vi "PLC.Debug.Simulator.vi"() -> ()   [LabVIEW 2016]
uses:
  Database/Database.Global.vi
  LowLevel/PLC.DataBlock.PLCchangeover.ctl
  LowLevel/PLC.DataBlock.PCchangeover.ctl
  LowLevel/PLC.DataBlock.PLCcheckstatus.ctl
  <vilib>/Utility/miscctls.llb/LVPointTypeDef.ctl
  LowLevel/PLC.DataBlock.PCcheckstatus.ctl
panel:
  in  "NewDataContinuous":bool caption="Status"
  out "_loop":i32(ring)=4
  in  "NewDataSingle":bool caption="Status"
  in  "NewDataComponentBAM":string="3000000" caption="Component BAM"
  in  "NewDataComponentHousing":string="2000000" caption="Component Housing"
  in  "NewDataProductSerial":string="1000000" caption="Product Serial"
  out "PLCcheckstatus":T1
  in  "CheckComponentSerial":string caption="Component Serial"
  out "PCcheckstatus":T2
  in  "CheckProductSerial":string caption="Product Serial"
  in  "CheckStatus":bool caption="Status"
  in  "CheckStation":i32(ring) caption="Station" items=["AS_010.01.A_cTCV", "AS_010.01.B_cTCV", "AS_010.01.C_cTCV", "AS_020.01.A_cTCV", "AS_030.01.A_cTCV", "AS_030.01.B_cTCV", "AS_040.01.A_cTCV", "AS_050.01.A_cTCV", "AS_060.01.A_cTCV", "AS_060.01.B_cTCV", "AS_060.01.C_cTCV", "AS_070.01.A_cTCV", "AS_070.02.A_cTCV", "AS_070.01.B_cTCV", "TB_071.01.A_cTCV", "AS_080.01.A_cTCV"]
  out "PCchangeover":T3 caption="AS_030.01.A_cTCV" {"TVH" format="%.3f"; "TVL" format="%.3f"; "TP" format="%.3f"}
  out "Variant.Refs":refnum<vi>[](array[refnum])
  in  "Variant BAM":u16(ring) caption="BAM" items=["", "9998887773"]
  in  "Variant Housing":u16(ring) caption="Housing" items=["", "9998887772"]
  in  "Variant ProdLine":u16(ring) caption="Main" items=["", "9998887770", "9998887771"]
  in  "Variant 15":u16(ring) caption="AS_080.01.A_cTCV" items=["", "9998887770", "9998887771"]
  in  "Variant 03":u16(ring) caption="AS_020.01.A_cTCV" items=["", "9998887770", "9998887771"]
  in  "Variant 14":u16(ring) caption="TB_071.01.A_cTCV" items=["", "9998887770", "9998887771"]
  in  "Variant 13":u16(ring) caption="AS_070.01.B_cTCV" items=["", "9998887770"]
  in  "Variant 12":u16(ring) caption="AS_070.02.A_cTCV" items=["", "9998887771"]
  in  "Variant 11":u16(ring) caption="AS_070.01.A_cTCV" items=["", "9998887770"]
  in  "Variant 10":u16(ring) caption="AS_060.01.C_cTCV" items=["", "9998887773"]
  in  "Variant 09":u16(ring) caption="AS_060.01.B_cTCV" items=["", "9998887773"]
  in  "Variant 08":u16(ring) caption="AS_060.01.A_cTCV" items=["", "9998887773"]
  in  "Variant 07":u16(ring) caption="AS_050.01.A_cTCV" items=["", "9998887770"]
  in  "Variant 06":u16(ring) caption="AS_040.01.A_cTCV" items=["", "9998887770", "9998887771"]
  in  "Variant 05":u16(ring) caption="AS_030.01.B_cTCV" items=["", "9998887772"]
  in  "Variant 04":u16(ring) caption="AS_030.01.A_cTCV" items=["", "9998887772"]
  in  "Variant 02":u16(ring) caption="AS_010.01.C_cTCV" items=["", "9998887770"]
  in  "Variant 01":u16(ring) caption="AS_010.01.B_cTCV" items=["", "9998887770", "9998887771"]
  in  "Variant 00":u16(ring) caption="AS_010.01.A_cTCV" items=["", "9998887770", "9998887771"]
  out "ChangeoverData":T3[](array[typedef]) {"TVH" format="%.3f"; "TVL" format="%.3f"; "TP" format="%.3f"}
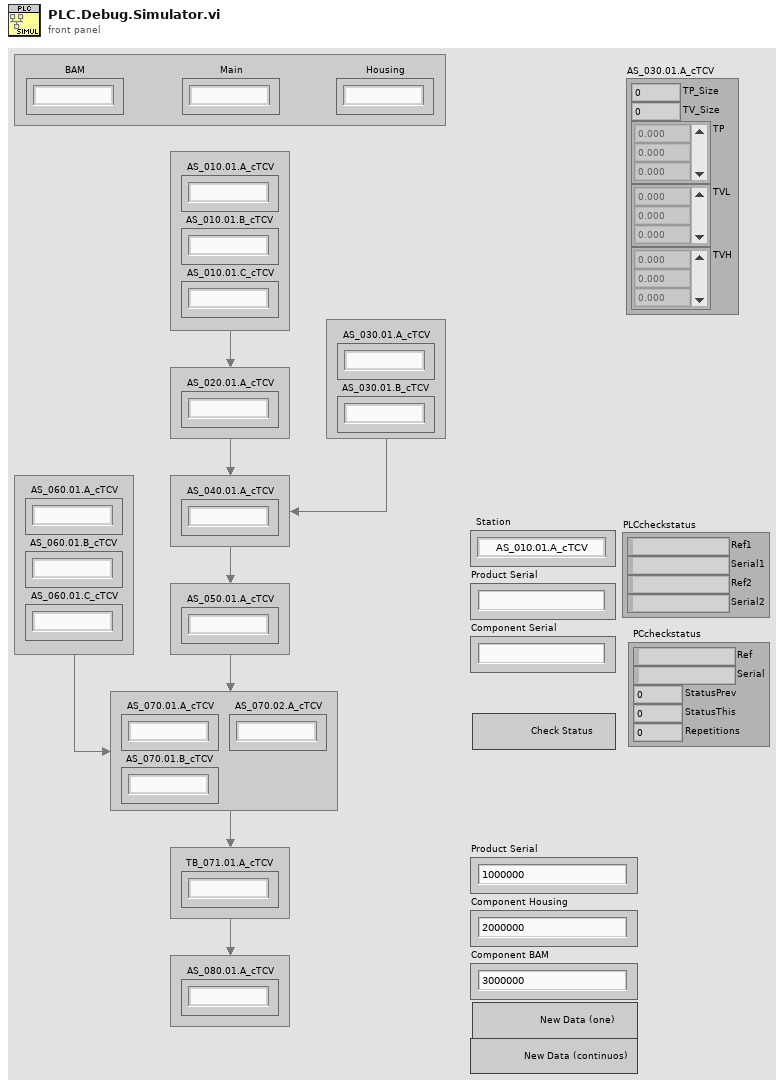
[diagram p1: front panel]
types:
  T1 = typedef "PLC.DataBlock.PLCcheckstatus.ctl" = cluster{"Ref1":string, "Serial1":string, "Ref2":string, "Serial2":string}
  T2 = typedef "PLC.DataBlock.PCcheckstatus.ctl" = cluster{"Ref":string, "Serial":string, "StatusPrev":i8, "StatusThis":i8, "Repetitions":u8}
  T3 = typedef "PLC.DataBlock.PCchangeover.ctl" = cluster{"TP_Size":u8, "TV_Size":u8, "TP":sgl[], "TVL":sgl[], "TVH":sgl[]}
  T4 = typedef "LVPointTypeDef.ctl" = cluster{"Horizontal":i16, "Vertical":i16}
  T5 = enum8{"Enabled", "Disabled", "Disabled and Grayed Out"}
  T6 = typedef "PLC.DataBlock.PLCchangeover.ctl" = cluster{"Ref":string}
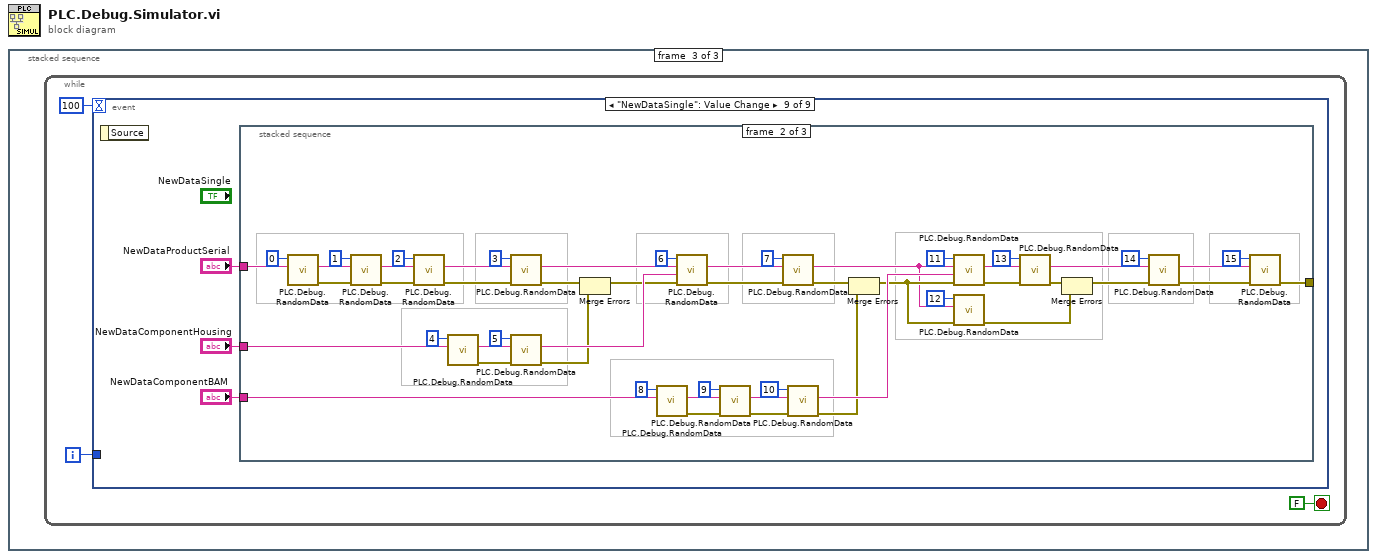
[diagram p0: block diagram]
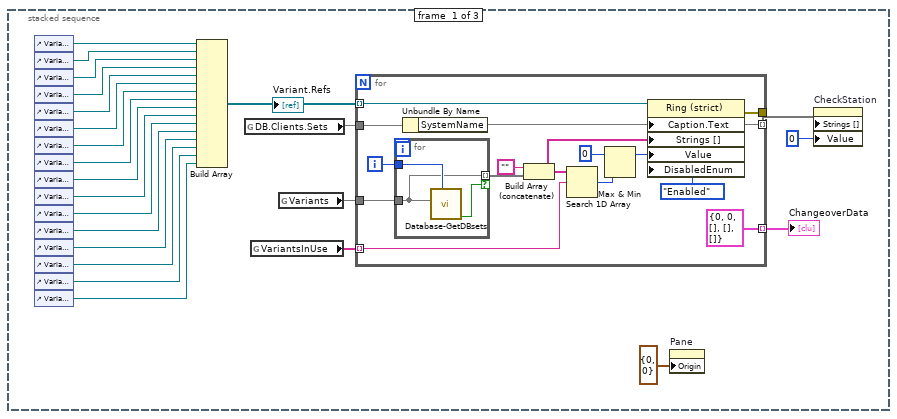
[diagram p2: hidden frame]
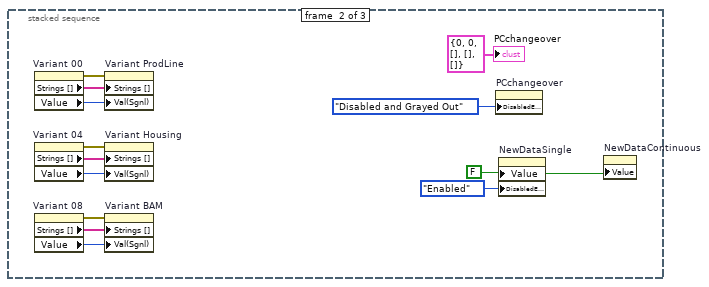
[diagram p3: hidden frame]
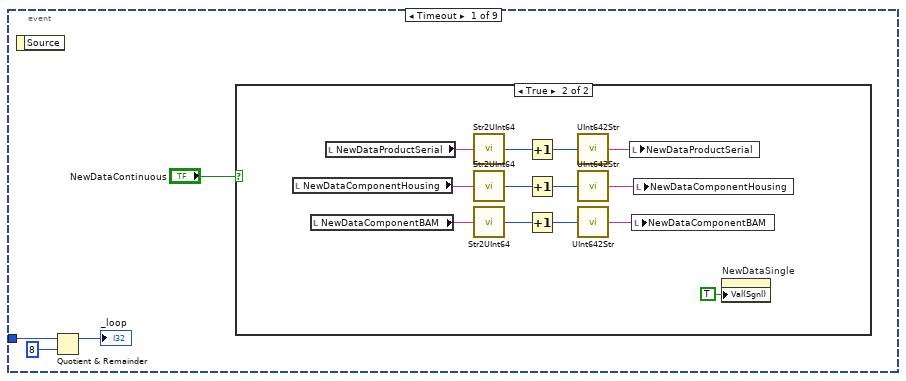
[diagram p4: hidden frame]
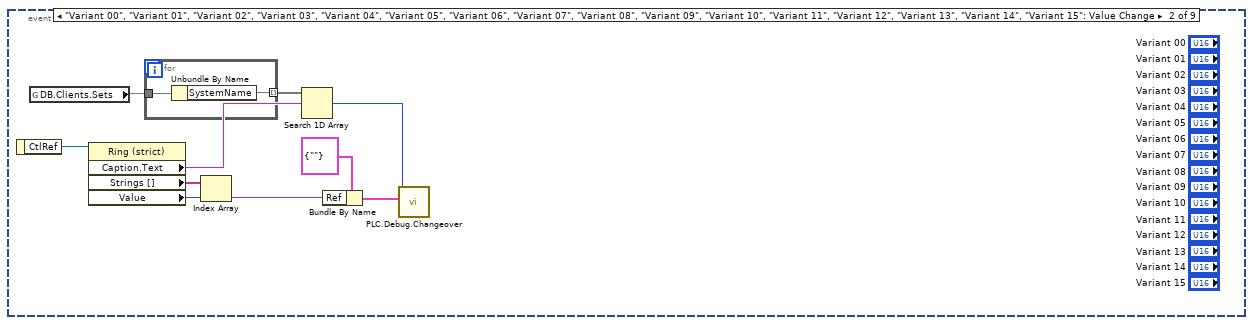
[diagram p6: hidden frame]
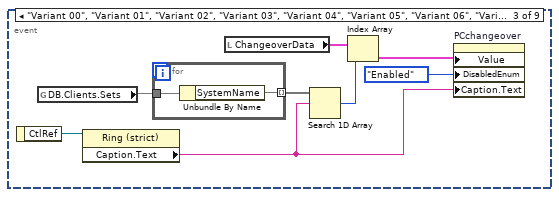
[diagram p7: hidden frame]
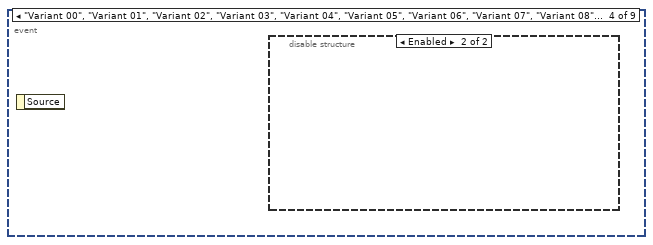
[diagram p8: hidden frame]
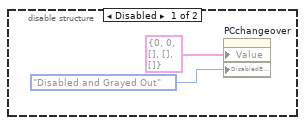
[diagram p9: hidden frame]
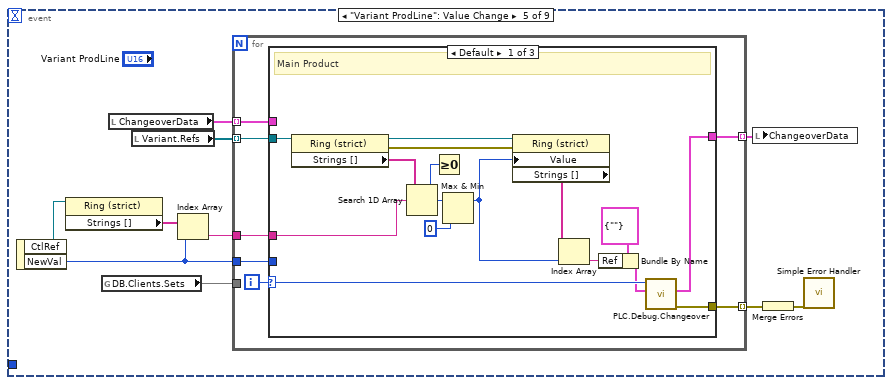
[diagram p10: hidden frame]
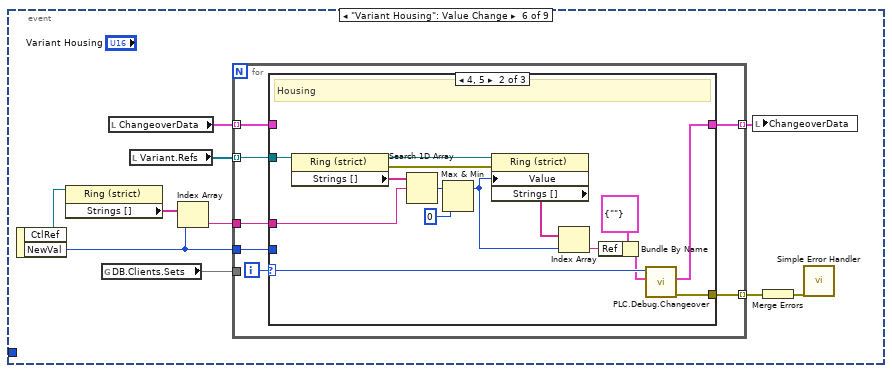
[diagram p13: hidden frame]
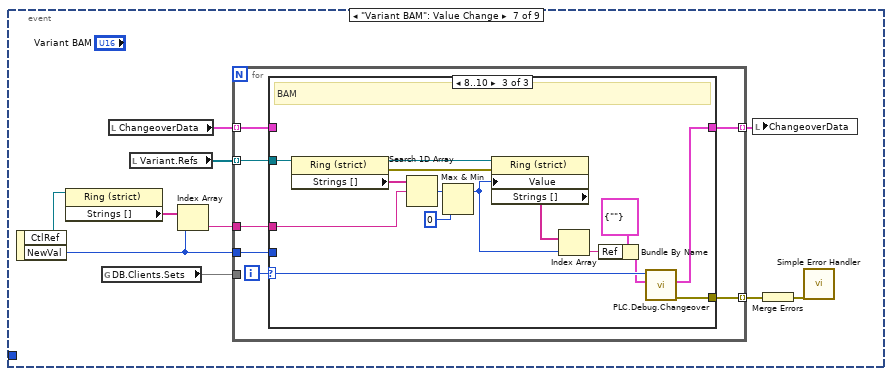
[diagram p16: hidden frame]
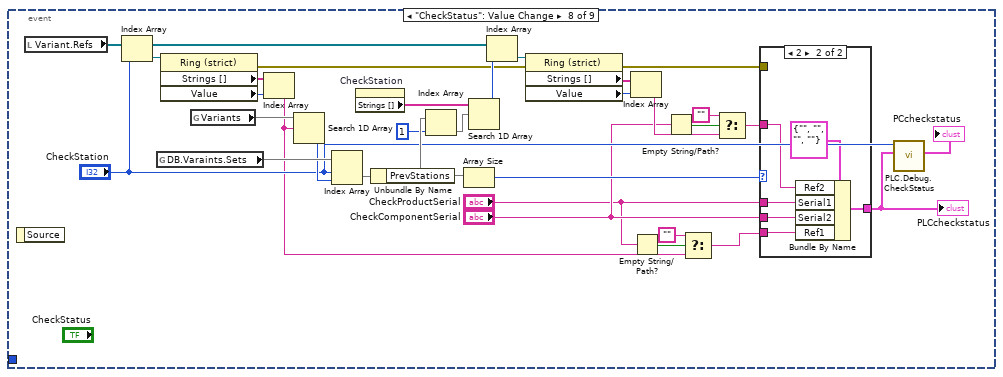
[diagram p19: hidden frame]
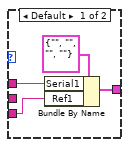
[diagram p20: hidden frame]
diagram:
  n1 = stacked-sequence {
    frame #0 {
      n2 = control-ref of="Variant 00"() -> (w7:refnum<vi>)
      n3 = control-ref of="Variant 01"() -> (w8:refnum<vi>)
      n4 = control-ref of="Variant 02"() -> (w9:refnum<vi>)
      n5 = control-ref of="Variant 03"() -> (w10:refnum<vi>)
      n6 = control-ref of="Variant 04"() -> (w11:refnum<vi>)
      n7 = control-ref of="Variant 05"() -> (w12:refnum<vi>)
      n8 = control-ref of="Variant 06"() -> (w13:refnum<vi>)
      n9 = control-ref of="Variant 07"() -> (w14:refnum<vi>)
      n10 = control-ref of="Variant 08"() -> (w15:refnum<vi>)
      n11 = control-ref of="Variant 09"() -> (w16:refnum<vi>)
      n12 = control-ref of="Variant 10"() -> (w17:refnum<vi>)
      n13 = control-ref of="Variant 11"() -> (w18:refnum<vi>)
      n14 = control-ref of="Variant 12"() -> (w19:refnum<vi>)
      n15 = control-ref of="Variant 13"() -> (w20:refnum<vi>)
      n16 = control-ref of="Variant 14"() -> (w21:refnum<vi>)
      n17 = control-ref of="Variant 15"() -> (w22:refnum<vi>)
      n18 = Build Array(w7, w8, w9, w10, w11, w12, w13, w14, w15, w16, w17, w18, w19, w20, w21, w22) -> (w6:refnum<vi>[])
      "Variant.Refs" <- w6
      n19 = global read "Database.Global.vi" "DB.Clients.Sets"() -> (w24)
      n20 = global read "Database.Global.vi" "VariantsInUse"() -> (w4:string[])
      n21 = global read "Database.Global.vi" "Variants"() -> (w23)
      n22 = for {
        tunnel: w24 -> [w37]
        tunnel: w23 -> [w39]
        tunnel: w6 -> [w33] mode=indexing
        tunnel: [w36] -> _
        tunnel: [T3 {"TP_Size"=0, "TV_Size"=0, "TP"=[], "TVL"=[], "TVH"=[]} ("PCchangeover")] -> w5 mode=indexing
        tunnel: w4 -> [w25] mode=indexing
        tunnel: [w26] -> w3 mode=indexing
        i -> [w38]
        n23 = for {
          tunnel: w39 -> [w41]
          tunnel: w38 -> [w42]
          tunnel: [w41] -> w35 mode=indexing if=w40
          n24 = call "Database-GetDBsets.vi"("Idx"=w42, "Variant"=w41) -> ("Found"=w40:bool)  [unwired: 5 in, 4 out]
        }
        n25 = Unbundle By Name(w37) -> ("SystemName"=w26)
        n26 = Build Array (concatenate)("", w35) -> (w28:string[])
        n27 = Search 1D Array(1D array=w28, element=w25) -> (index of element=w31:i32)  [unwired: 1 in]
        n28 = Max & Min(x=0 ("Value"), y=w31) -> (max(x,y)=w29:i32)  [unwired: 1 out]
        n29 = property class="Ring (strict)"(reference=w33, "Caption.Text"=w26, "Strings []"=w28, "Value"=w29, "DisabledEnum"=T5."Enabled" ("Disabled")) -> (error out=w36:errorcluster)  [unwired: 1 in, 1 out]
      }
      "ChangeoverData" <- w5
      n30 = property on="Pane" class="Pane"("Origin"=T4 {"Horizontal"=0, "Vertical"=0}) -> ()  [unwired: 2 in, 2 out]
      n31 = property on="CheckStation" class="Ring (strict)"("Strings []"=w3, "Value"=0) -> ()  [unwired: 2 in, 2 out]
    }
    frame #1 {
      w43 = FALSE ("NewDataSingle")
      n32 = property on="Variant 00" class="Ring (strict)"() -> (error out=w52:errorcluster, "Strings []"=w55:string[], "Value"=w47:u16)  [unwired: 2 in, 1 out]
      n33 = property on="Variant 04" class="Ring (strict)"() -> (error out=w51:errorcluster, "Strings []"=w54:string[], "Value"=w48:u16)  [unwired: 2 in, 1 out]
      n34 = property on="Variant 08" class="Ring (strict)"() -> (error out=w50:errorcluster, "Strings []"=w53:string[], "Value"=w49:u16)  [unwired: 2 in, 1 out]
      n35 = property on="Variant ProdLine" class="Ring (strict)"(error in=w52, "Strings []"=w55, "Val(Sgnl)"=w47) -> ()  [unwired: 1 in, 2 out]
      n36 = property on="Variant Housing" class="Ring (strict)"(error in=w51, "Strings []"=w54, "Val(Sgnl)"=w48) -> ()  [unwired: 1 in, 2 out]
      n37 = property on="Variant BAM" class="Ring (strict)"(error in=w50, "Strings []"=w53, "Val(Sgnl)"=w49) -> ()  [unwired: 1 in, 2 out]
      n38 = property on="PCchangeover" class="Clust (strict)"("DisabledEnum"=T5."Disabled and Grayed Out" ("Disabled")) -> ()  [unwired: 2 in, 2 out]
      n39 = property on="NewDataSingle" class="Bool (strict)"("Value"=w43, "DisabledEnum"=T5."Enabled" ("Disabled")) -> ()  [unwired: 2 in, 2 out]
      n40 = property on="NewDataContinuous" class="Bool (strict)"("Value"=w43) -> ()  [unwired: 2 in, 2 out]
      "PCchangeover" <- T3 {"TP_Size"=0, "TV_Size"=0, "TP"=[], "TVL"=[], "TVH"=[]} ("PCchangeover")
    }
    frame #2 {
      n41 = while {
        i -> [w56]
        stop <- FALSE stop-if-true
        n42 = event shown="[8] \"NewDataSingle\": Value Change" {
          selector: _ -> [_ _ _ _ _ _ _ _ _]
          dyn-events: _ -> [_ _ _ _ _ _ _ _ _]
          timeout: 100 -> [_ _ _ _ _ _ _ _ _]
          tunnel: w56 -> [w60 _ _ _ _ _ _ _ _]
          event Timeout {
            n43 = event-data() -> ()  [unwired: 1 in, 1 out]
            n44 = Quotient & Remainder(x=w60, y=8) -> (x-y*floor(x/y)=→"_loop":i32)  [unwired: 1 out]
            n45 = case shown="True" "NewDataContinuous" {
              frame False {
              }
              frame True {
                n46 = local read "NewDataComponentHousing"() -> (w70:string)
                n47 = local read "NewDataComponentBAM"() -> (w65:string)
                n48 = local read "NewDataProductSerial"() -> (w73:string)
                n49 = call "Str2UInt64.vi"("string"=w73) -> ("Numeric"=w74:u64)
                n50 = call "Str2UInt64.vi"("string"=w70) -> ("Numeric"=w69:u64)
                n51 = call "Str2UInt64.vi"("string"=w65) -> ("Numeric"=w66:u64)
                n52 = Increment(x=w74) -> (x+1=w72:u64)
                n53 = Increment(x=w69) -> (x+1=w71:u64)
                n54 = Increment(x=w66) -> (x+1=w64:u64)
                n55 = call "UInt642Str.vi"("Numeric"=w72) -> ("string"=w75:string)
                n56 = call "UInt642Str.vi"("Numeric"=w71) -> ("string"=w68:string)
                n57 = call "UInt642Str.vi"("Numeric"=w64) -> ("string"=w67:string)
                n58 = local write "NewDataProductSerial"(w75) -> ()
                n59 = local write "NewDataComponentBAM"(w67) -> ()
                n60 = local write "NewDataComponentHousing"(w68) -> ()
                n61 = property on="NewDataSingle" class="Bool (strict)"("Val(Sgnl)"=TRUE ("Value (Signaling)")) -> ()  [unwired: 2 in, 2 out]
              }
            }
          }
          event "Variant 00", "Variant 01", "Variant 02", "Variant 03", "Variant 04", "Variant 05", "Variant 06", "Variant 07", "Variant 08", "Variant 09", "Variant 10", "Variant 11", "Variant 12", "Variant 13", "Variant 14", "Variant 15": Value Change {
            n62 = event-data() -> ("CtlRef"=w85:refnum<vi>)  [unwired: 1 in]
            n63 = global read "Database.Global.vi" "DB.Clients.Sets"() -> (w79)
            n64 = property class="Ring (strict)"(reference=w85) -> ("Caption.Text"=w77:string, "Strings []"=w82:string[], "Value"=w83:u16)  [unwired: 1 in, 2 out]
            n65 = for {
              tunnel: w79 -> [w87]
              tunnel: [w86] -> w78 mode=indexing
              n66 = Unbundle By Name(w87) -> ("SystemName"=w86)
            }
            n67 = Index Array(array=w82, index=w83) -> (element=w81:string)
            n68 = Search 1D Array(1D array=w78, element=w77) -> (index of element=w76:i32)  [unwired: 1 in]
            n69 = Bundle By Name(cluster=T6 {"Ref"=""} ("PLCchangeover"), "Ref"=w81) -> (w80:T6)
            n70 = call "PLC.Debug.Changeover.vi"("PLCchangeover"=w80, "Idx"=w76) -> ()  [unwired: 8 in, 2 out]
          }
          event "Variant 00", "Variant 01", "Variant 02", "Variant 03", "Variant 04", "Variant 05", "Variant 06", "Variant 07", "Variant 08", "Variant 09", "Variant 10", "Variant 12", "Variant 13", "Variant 14", "Variant 15": Mouse Enter {
            n71 = event-data() -> ("CtlRef"=w95:refnum<vi>)  [unwired: 1 in]
            n72 = global read "Database.Global.vi" "DB.Clients.Sets"() -> (w92)
            n73 = property class="Ring (strict)"(reference=w95) -> ("Caption.Text"=w88:string)  [unwired: 1 in, 2 out]
            n74 = for {
              tunnel: w92 -> [w97]
              tunnel: [w96] -> w91 mode=indexing
              n75 = Unbundle By Name(w97) -> ("SystemName"=w96)
            }
            n76 = local read "ChangeoverData"() -> (w94:T3[])
            n77 = Search 1D Array(1D array=w91, element=w88) -> (index of element=w90:i32)  [unwired: 1 in]
            n78 = Index Array(array=w94, index=w90) -> (element=w93:T3)
            n79 = property on="PCchangeover" class="Clust (strict)"("Value"=w93, "DisabledEnum"=T5."Enabled" ("Disabled"), "Caption.Text"=w88) -> ()  [unwired: 2 in, 2 out]
          }
          event "Variant 00", "Variant 01", "Variant 02", "Variant 03", "Variant 04", "Variant 05", "Variant 06", "Variant 07", "Variant 08", "Variant 09", "Variant 10", "Variant 11", "Variant 12", "Variant 13", "Variant 14", "Variant 15": Mouse Leave {
            n80 = event-data() -> ()  [unwired: 1 in, 1 out]
            n81 = disable-structure shown="Enabled" {
              frame Disabled {
                n82 = property on="PCchangeover" class="Clust (strict)"("Value"=T3 {"TP_Size"=0, "TV_Size"=0, "TP"=[], "TVL"=[], "TVH"=[]} ("PCchangeover"), "DisabledEnum"=T5."Disabled and Grayed Out" ("Disabled")) -> ()  [unwired: 2 in, 2 out]
              }
              frame Enabled {
              }
            }
          }
          event "Variant ProdLine": Value Change {
            n83 = event-data() -> ("CtlRef"=w101:refnum<vi>, "NewVal"=w102:u16)  [unwired: 1 in]
            n84 = property class="Ring (strict)"(reference=w101) -> ("Strings []"=w103:string[])  [unwired: 1 in, 2 out]
            n85 = global read "Database.Global.vi" "DB.Clients.Sets"() -> (w109)
            n86 = local read "ChangeoverData"() -> (w105:T3[])
            n87 = local read "Variant.Refs"() -> (w106:refnum<vi>[])
            n88 = Index Array(array=w103, index=w102) -> (element=w100:string)
            n89 = for {
              tunnel: w109 -> [_]
              tunnel: w106 -> [w111] mode=indexing
              tunnel: w102 -> [w115]
              tunnel: [w114] -> w108 mode=indexing
              tunnel: w105 -> [w113] mode=indexing
              tunnel: [w112] -> w104 mode=indexing
              tunnel: w100 -> [w110]
              i -> [w116]
              n90 = case shown="Default" w116 {
                selector: w116 -> [w129 _ _]
                tunnel: w111 -> [w125 _ _]
                tunnel: w115 -> [_ _ _]
                tunnel: [w127 _ _] -> w114
                tunnel: w113 -> [_ w132 w133]
                tunnel: [w126 w132 w133] -> w112
                tunnel: w110 -> [w122 _ _]
                frame Default {
                  # "Main Product"
                  n91 = property class="Ring (strict)"(reference=w125) -> (reference out=w124:refnum<vi>, error out=w120:errorcluster, "Strings []"=w123:string[])  [unwired: 1 in]
                  n92 = Search 1D Array(1D array=w123, element=w122) -> (index of element=w117:i32)  [unwired: 1 in]
                  n93 = Greater Or Equal To 0?(x=w117) -> ()  [unwired: 1 out]
                  n94 = Max & Min(x=w117, y=0) -> (max(x,y)=w118:i32)  [unwired: 1 out]
                  n95 = property class="Ring (strict)"(reference=w124, error in=w120, "Value"=w118) -> ("Strings []"=w119:string[])  [unwired: 2 out]
                  n96 = Index Array(array=w119, index=w118) -> (element=w130:string)
                  n97 = Bundle By Name(cluster=T6 {"Ref"=""} ("PLCchangeover"), "Ref"=w130) -> (w128:T6)
                  n98 = call "PLC.Debug.Changeover.vi"("PLCchangeover"=w128, "Idx"=w129) -> ("error out"=w127:errorcluster, "PCchangeover"=w126:T3)  [unwired: 8 in]
                }
                frame 4, 5 {
                  # "Housing"
                }
                frame 8..10 {
                  # "BAM"
                }
              }
            }
            n99 = local write "ChangeoverData"(w104) -> ()
            n100 = Merge Errors(w108) -> (w107:errorcluster)
            n101 = call <vilib>:"Simple Error Handler.vi"("error in (no error)"=w107) -> ()  [unwired: 4 in, 5 out]
          }
          event "Variant Housing": Value Change {
            n102 = event-data() -> ("CtlRef"=w135:refnum<vi>, "NewVal"=w136:u16)  [unwired: 1 in]
            n103 = property class="Ring (strict)"(reference=w135) -> ("Strings []"=w137:string[])  [unwired: 1 in, 2 out]
            n104 = global read "Database.Global.vi" "DB.Clients.Sets"() -> (w143)
            n105 = local read "ChangeoverData"() -> (w139:T3[])
            n106 = local read "Variant.Refs"() -> (w140:refnum<vi>[])
            n107 = Index Array(array=w137, index=w136) -> (element=w134:string)
            n108 = for {
              tunnel: w143 -> [_]
              tunnel: w140 -> [w145] mode=indexing
              tunnel: w136 -> [w149]
              tunnel: [w148] -> w142 mode=indexing
              tunnel: w139 -> [w147] mode=indexing
              tunnel: [w146] -> w138 mode=indexing
              tunnel: w134 -> [w144]
              i -> [w150]
              n109 = case shown="4, 5" w150 {
                selector: w150 -> [_ w164 _]
                tunnel: w145 -> [_ w160 _]
                tunnel: w149 -> [_ _ _]
                tunnel: [_ w162 _] -> w148
                tunnel: w147 -> [w151 _ w167]
                tunnel: [w151 w161 w167] -> w146
                tunnel: w144 -> [_ w157 _]
                frame Default {
                  # "Main Product"
                }
                frame 4, 5 {
                  # "Housing"
                  n110 = property class="Ring (strict)"(reference=w160) -> (reference out=w159:refnum<vi>, error out=w154:errorcluster, "Strings []"=w158:string[])  [unwired: 1 in]
                  n111 = Search 1D Array(1D array=w158, element=w157) -> (index of element=w156:i32)  [unwired: 1 in]
                  n112 = Max & Min(x=w156, y=0) -> (max(x,y)=w152:i32)  [unwired: 1 out]
                  n113 = property class="Ring (strict)"(reference=w159, error in=w154, "Value"=w152) -> ("Strings []"=w153:string[])  [unwired: 2 out]
                  n114 = Index Array(array=w153, index=w152) -> (element=w165:string)
                  n115 = Bundle By Name(cluster=T6 {"Ref"=""} ("PLCchangeover"), "Ref"=w165) -> (w163:T6)
                  n116 = call "PLC.Debug.Changeover.vi"("PLCchangeover"=w163, "Idx"=w164) -> ("error out"=w162:errorcluster, "PCchangeover"=w161:T3)  [unwired: 8 in]
                }
                frame 8..10 {
                  # "BAM"
                }
              }
            }
            n117 = local write "ChangeoverData"(w138) -> ()
            n118 = Merge Errors(w142) -> (w141:errorcluster)
            n119 = call <vilib>:"Simple Error Handler.vi"("error in (no error)"=w141) -> ()  [unwired: 4 in, 5 out]
          }
          event "Variant BAM": Value Change {
            n120 = event-data() -> ("CtlRef"=w169:refnum<vi>, "NewVal"=w170:u16)  [unwired: 1 in]
            n121 = property class="Ring (strict)"(reference=w169) -> ("Strings []"=w171:string[])  [unwired: 1 in, 2 out]
            n122 = global read "Database.Global.vi" "DB.Clients.Sets"() -> (w177)
            n123 = local read "ChangeoverData"() -> (w173:T3[])
            n124 = local read "Variant.Refs"() -> (w174:refnum<vi>[])
            n125 = Index Array(array=w171, index=w170) -> (element=w168:string)
            n126 = for {
              tunnel: w177 -> [_]
              tunnel: w174 -> [w179] mode=indexing
              tunnel: w170 -> [w183]
              tunnel: [w182] -> w176 mode=indexing
              tunnel: w173 -> [w181] mode=indexing
              tunnel: [w180] -> w172 mode=indexing
              tunnel: w168 -> [w178]
              i -> [w184]
              n127 = case shown="8..10" w184 {
                selector: w184 -> [_ _ w199]
                tunnel: w179 -> [_ _ w195]
                tunnel: w183 -> [_ _ _]
                tunnel: [_ _ w197] -> w182
                tunnel: w181 -> [w185 w186 _]
                tunnel: [w185 w186 w196] -> w180
                tunnel: w178 -> [_ _ w192]
                frame Default {
                  # "Main Product"
                }
                frame 4, 5 {
                  # "Housing"
                }
                frame 8..10 {
                  # "BAM"
                  n128 = property class="Ring (strict)"(reference=w195) -> (reference out=w194:refnum<vi>, error out=w189:errorcluster, "Strings []"=w193:string[])  [unwired: 1 in]
                  n129 = Search 1D Array(1D array=w193, element=w192) -> (index of element=w191:i32)  [unwired: 1 in]
                  n130 = Max & Min(x=w191, y=0) -> (max(x,y)=w187:i32)  [unwired: 1 out]
                  n131 = property class="Ring (strict)"(reference=w194, error in=w189, "Value"=w187) -> ("Strings []"=w188:string[])  [unwired: 2 out]
                  n132 = Index Array(array=w188, index=w187) -> (element=w200:string)
                  n133 = Bundle By Name(cluster=T6 {"Ref"=""} ("PLCchangeover"), "Ref"=w200) -> (w198:T6)
                  n134 = call "PLC.Debug.Changeover.vi"("PLCchangeover"=w198, "Idx"=w199) -> ("error out"=w197:errorcluster, "PCchangeover"=w196:T3)  [unwired: 8 in]
                }
              }
            }
            n135 = local write "ChangeoverData"(w172) -> ()
            n136 = Merge Errors(w176) -> (w175:errorcluster)
            n137 = call <vilib>:"Simple Error Handler.vi"("error in (no error)"=w175) -> ()  [unwired: 4 in, 5 out]
          }
          event "CheckStatus": Value Change {
            n138 = event-data() -> ()  [unwired: 1 in, 1 out]
            n139 = local read "Variant.Refs"() -> (w214:refnum<vi>[])
            n140 = Index Array(array=w214, index="CheckStation") -> (element=w233:refnum<vi>)
            n141 = global read "Database.Global.vi" "DB.Varaints.Sets"() -> (w230)
            n142 = property class="Ring (strict)"(reference=w233) -> (error out=w213:errorcluster, "Strings []"=w231:string[], "Value"=w232:u16)  [unwired: 1 in, 1 out]
            n143 = global read "Database.Global.vi" "Variants"() -> (w222)
            n144 = Index Array(array=w231, index=w232) -> (element=w210:string)
            n145 = Search 1D Array(1D array=w222, element=w210) -> (index of element=w229:i32)  [unwired: 1 in]
            n146 = Index Array(array=w230, index (row)="CheckStation", index (col)=w229) -> (element=w228)
            n147 = property on="CheckStation" class="Ring (strict)"() -> ("Strings []"=w226:string[])  [unwired: 2 in, 2 out]
            n148 = Unbundle By Name(w228) -> ("PrevStations"=w225)
            n149 = Index Array(array=w225, index=1) -> (element=w220)
            n150 = Array Size(array=w225) -> (size(s)=w227:i32)
            n151 = Search 1D Array(1D array=w226, element=w220) -> (index of element=w223:i32)  [unwired: 1 in]
            n152 = Index Array(array=w214, index=w223) -> (element=w216:refnum<vi>)
            n153 = property class="Ring (strict)"(reference=w216, error in=w213) -> (error out=w215:errorcluster, "Strings []"=w219:string[], "Value"=w218:u16)  [unwired: 1 out]
            n154 = Index Array(array=w219, index=w218) -> (element=w205:string)
            n155 = Empty String/Path?(string/path="CheckProductSerial") -> (empty?=w211:bool)
            n156 = Empty String/Path?(string/path="CheckComponentSerial") -> (empty?=w207:bool)
            n157 = Select(t="", s=w211, f=w210) -> (s? t:f=w208:string)
            n158 = Select(t="", s=w207, f=w205) -> (s? t:f=w204:string)
            n159 = case shown="2" w227 {
              tunnel: [w237 w243] -> w221
              tunnel: w208 -> [w236 w242]
              tunnel: "CheckProductSerial" -> [w235 w241]
              tunnel: "CheckComponentSerial" -> [_ w240]
              tunnel: w204 -> [_ w238]
              tunnel: w215 -> [_ _]
              frame Default {
                n160 = Bundle By Name(cluster=T1 {"Ref1"="", "Serial1"="", "Ref2"="", "Serial2"=""} ("PLCcheckstatus"), "Serial1"=w235, "Ref1"=w236) -> (w237:T1)
              }
              frame 2 {
                n161 = Bundle By Name(cluster=T1 {"Ref1"="", "Serial1"="", "Ref2"="", "Serial2"=""} ("PLCcheckstatus"), "Ref2"=w238, "Serial1"=w241, "Serial2"=w240, "Ref1"=w242) -> (w243:T1)
              }
            }
            "PLCcheckstatus" <- w221
            n162 = call "PLC.Debug.CheckStatus.vi"("PLCcheckstatus"=w221, "Idx"="CheckStation") -> ("PCcheckstatus"=→"PCcheckstatus":T2)  [unwired: 8 in, 1 out]
          }
          event "NewDataSingle": Value Change {
            n163 = event-data() -> ()  [unwired: 1 in, 1 out]
            n164 = stacked-sequence {
              tunnel: "NewDataComponentHousing" -> [_ w286 _]
              tunnel: "NewDataComponentBAM" -> [_ w285 _]
              tunnel: "NewDataProductSerial" -> [_ w249 _]
              tunnel: [_ w250 _] -> _
              frame #0 {
                n165 = property on="NewDataSingle" class="Bool (strict)"("Value"=TRUE ("NewDataSingle"), "DisabledEnum"=T5."Disabled and Grayed Out" ("Disabled")) -> ()  [unwired: 2 in, 2 out]
              }
              frame #1 {
                n166 = call "PLC.Debug.RandomData.vi"("Serial.Product"=w249, "Idx"=0) -> ("error out"=w281:errorcluster)  [unwired: 9 in]
                n167 = call "PLC.Debug.RandomData.vi"("error in (no error)"=w281, "Serial.Product"=w249, "Idx"=1) -> ("error out"=w280:errorcluster)  [unwired: 8 in]
                n168 = call "PLC.Debug.RandomData.vi"("error in (no error)"=w280, "Serial.Product"=w249, "Idx"=2) -> ("error out"=w278:errorcluster)  [unwired: 8 in]
                n169 = call "PLC.Debug.RandomData.vi"("Serial.Product"=w286, "Idx"=4) -> ("error out"=w277:errorcluster)  [unwired: 9 in]
                n170 = call "PLC.Debug.RandomData.vi"("error in (no error)"=w278, "Serial.Product"=w249, "Idx"=3) -> ("error out"=w273:errorcluster)  [unwired: 8 in]
                n171 = call "PLC.Debug.RandomData.vi"("error in (no error)"=w277, "Serial.Product"=w286, "Idx"=5) -> ("error out"=w268:errorcluster)  [unwired: 8 in]
                n172 = Merge Errors(w273, w268) -> (w267:errorcluster)
                n173 = call "PLC.Debug.RandomData.vi"("Serial.Product"=w285, "Idx"=8) -> ("error out"=w264:errorcluster)  [unwired: 9 in]
                n174 = call "PLC.Debug.RandomData.vi"("error in (no error)"=w267, "Serial.Component"=w286, "Serial.Product"=w249, "Idx"=6) -> ("error out"=w271:errorcluster)  [unwired: 7 in]
                n175 = call "PLC.Debug.RandomData.vi"("error in (no error)"=w264, "Serial.Product"=w285, "Idx"=9) -> ("error out"=w262:errorcluster)  [unwired: 8 in]
                n176 = call "PLC.Debug.RandomData.vi"("error in (no error)"=w271, "Serial.Product"=w249, "Idx"=7) -> ("error out"=w269:errorcluster)  [unwired: 8 in]
                n177 = call "PLC.Debug.RandomData.vi"("error in (no error)"=w262, "Serial.Product"=w285, "Idx"=10) -> ("error out"=w261:errorcluster)  [unwired: 8 in]
                n178 = Merge Errors(w269, w261) -> (w259:errorcluster)
                n179 = call "PLC.Debug.RandomData.vi"("error in (no error)"=w259, "Serial.Component"=w285, "Serial.Product"=w249, "Idx"=11) -> ("error out"=w257:errorcluster)  [unwired: 7 in]
                n180 = call "PLC.Debug.RandomData.vi"("error in (no error)"=w259, "Serial.Product"=w249, "Idx"=12) -> ("error out"=w255:errorcluster)  [unwired: 8 in]
                n181 = call "PLC.Debug.RandomData.vi"("error in (no error)"=w257, "Serial.Product"=w249, "Idx"=13) -> ("error out"=w256:errorcluster)  [unwired: 8 in]
                n182 = Merge Errors(w256, w255) -> (w253:errorcluster)
                n183 = call "PLC.Debug.RandomData.vi"("error in (no error)"=w253, "Serial.Product"=w249, "Idx"=14) -> ("error out"=w251:errorcluster)  [unwired: 8 in]
                n184 = call "PLC.Debug.RandomData.vi"("error in (no error)"=w251, "Serial.Product"=w249, "Idx"=15) -> ("error out"=w250:errorcluster)  [unwired: 8 in]
              }
              frame #2 {
                n185 = property on="NewDataSingle" class="Bool (strict)"("Value"=FALSE ("NewDataSingle"), "DisabledEnum"=T5."Enabled" ("Disabled")) -> ()  [unwired: 2 in, 2 out]
              }
            }
          }
        }
      }
    }
  }
